vi "dfd_Validate Params for Comb Design by f0.vi"(6 "fs [Hz]":dbl=1.0 format="%.2f", 7 "filter type":T1(ring), 8 "error in (no error)":errorcluster, 9 "bandwidth [Hz]":dbl=0.2 format="%.2f", 10 "Ab [dB]":dbl=3.010299956639812 format="%#.6g", 11 "f0 [Hz]":dbl=0.1 format="%.2f") -> (0 "error out":errorcluster, 1 "normalized BW [rad/s]":dbl format="%.2f", 2 "dup Ab [dB]":dbl format="%.2f", 3 "dup order":i32)   [LabVIEW 2017, in "NI_DigFilter_Design.lvlib"]
uses:
  <vilib>/addons/Digital Filter Design/NI_DigFilter_Design.lvlib
  <vilib>/addons/Digital Filter Design/_Misc.llb/dfd_Error Handlers (Multiple).vi
  <vilib>/addons/Digital Filter Design/_Misc.llb/dfd_X Equal Y (Scalar).vi
  <vilib>/addons/Digital Filter Design/NI_DigFilterLicensed.lvlib
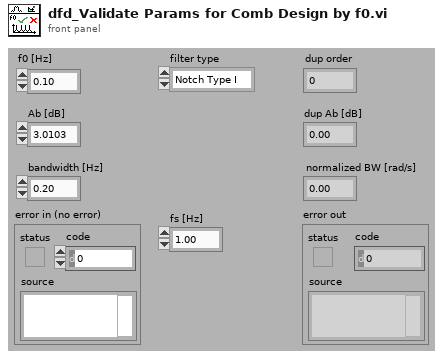
[diagram p1: front panel]
types:
  T1 = enum16{"Notch Type I", "Notch Type II", "Peak Type I", "Peak Type II"}
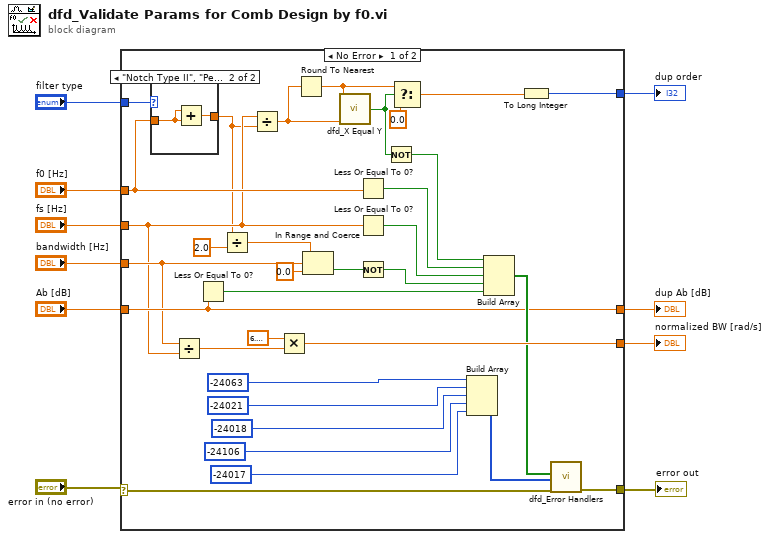
[diagram p0: block diagram]
diagram:
  n1 = case shown="No Error" "error in (no error)" {
    selector: "error in (no error)" -> [w39 w47]
    tunnel: [w38 _] -> w10
    tunnel: "Ab [dB]" -> [w38 _]
    tunnel: "bandwidth [Hz]" -> [w25 _]
    tunnel: [w43 _] -> w7
    tunnel: "f0 [Hz]" -> [w31 _]
    tunnel: [w42 w47] -> w6
    tunnel: [w26 _] -> w3
    tunnel: "fs [Hz]" -> [w13 _]
    tunnel: "filter type" -> [w32 _]
    frame No Error {
      n2 = case shown="\"Notch Type II\", \"Peak Type II\"" w32 {
        tunnel: w31 -> [w44 w45]
        tunnel: [w44 w46] -> w12
        frame "Notch Type I", "Peak Type I", Default {
        }
        frame "Notch Type II", "Peak Type II" {
          n3 = Add(x=w45, y=w45) -> (x+y=w46:dbl)
        }
      }
      n4 = Divide(x=w25, y=w13) -> (x/y=w33:dbl)
      n5 = Less Or Equal To 0?(x=w38) -> (x <= 0?=w35:bool)
      n6 = Divide(x=w12, y=2.0) -> (x/y=w23:dbl)
      n7 = Divide(x=w13, y=w12) -> (x/y=w27:dbl)
      n8 = Multiply(x=6.283185307179586, y=w33) -> (x*y=w43:dbl)
      n9 = Round To Nearest(number=w27) -> (nearest integer value=w28:dbl)
      n10 = In Range and Coerce(upper limit=w23, x=w25, lower limit=0.0) -> (In Range?=w22:bool)  [unwired: 1 out]
      n11 = call-poly <vilib>:"dfd_X Equal Y.vi"("x"=w28, "y"=w27) -> ("x = y?"=w14:bool)  [unwired: 1 in, 4 out]
      n12 = Less Or Equal To 0?(x=w31) -> (x <= 0?=w34:bool)
      n13 = Less Or Equal To 0?(x=w13) -> (x <= 0?=w15:bool)
      n14 = Not(x=w22) -> (.not. x?=w21:bool)
      n15 = Not(x=w14) -> (.not. x?=w11:bool)
      n16 = Select(t=w28, s=w14, f=0.0) -> (s? t:f=w30:dbl)
      n17 = Build Array(-24063 ("ERR_COMB_F0_WRONG"), -24021 ("ERR_FREQ_RANGE_WRONG"), -24018 ("ERR_FS_LE_ZERO"), -24106 ("ERR_COMB_BW_BYF0_RANGE_WRONG"), -24017 ("ERR_dB_LE_ZERO")) -> (w40:i32[])
      n18 = Build Array(w11, w34, w15, w21, w35) -> (w41:bool[])
      n19 = To Long Integer(number=w30) -> (32bit integer=w26:i32)
      n20 = call-poly <vilib>:"dfd_Error Handlers.vi"("error in (no error)"=w39, "error sources"=w40, "condition failed?"=w41) -> ("error out"=w42:errorcluster)  [unwired: 8 out]
    }
    frame Error {
    }
  }
  "dup Ab [dB]" <- w10
  "normalized BW [rad/s]" <- w7
  "error out" <- w6
  "dup order" <- w3
